vi "PH_ImageOperator.write PSDB Images data.vi"(0 "i ref in":refnum<vi>, 5 "error in":errorcluster) -> (14 "i ref out":refnum<vi>, 16 "Images Image data":T1[](array[typedef]), 17 "Images Boolean data":T3[](array[typedef]), 19 "error out":errorcluster)   [LabVIEW 2014, in "PH_ImageOperator.lvlib"]
uses:
  PH_ImageOperator.lvlib
  PH_Basics/PH_PSDBWriter/PH_PSDBWriter.Boolean dataset.ctl
  PH_Basics/PH_PSDBWriter/PH_PSDBWriter.Image dataset.ctl
  <vilib>/vision/Image Controls.llb/IMAQ Image.ctl
  <vilib>/vision/NI_Vision_Development_Module.lvlib
  PH_Basics/PH_PSDBWriter/PH_PSDBWriter.lvlib
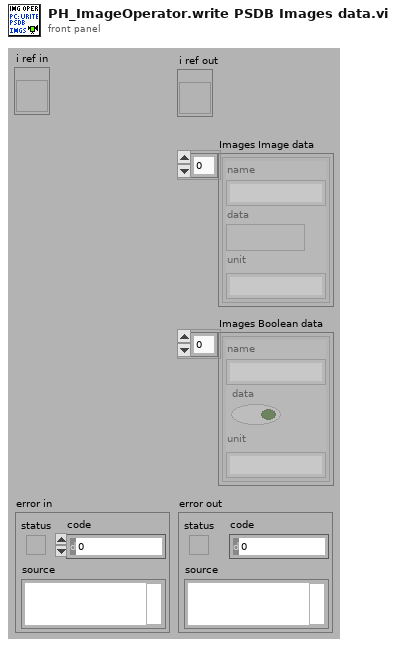
[diagram p1: front panel]
types:
  T1 = typedef "PH_PSDBWriter.lvlib/PH_PSDBWriter.Image dataset.ctl" = cluster{"name":string, "data":T2, "unit":string}
  T2 = typedef "IMAQ Image.ctl" = refnum<image>
  T3 = typedef "PH_PSDBWriter.lvlib/PH_PSDBWriter.Boolean dataset.ctl" = cluster{"name":string, "data":bool, "unit":string}
  T4 = typedef "Image Type" = u32
  T5 = typedef "PH_ImageOperator.lvlib/PH_ImageOperator.i attribute.ctl" = cluster{"GUI Refs":cluster{"Delete":refnum<vi>, "Calibration status":refnum<vi>, "BI subtracted":refnum<vi>, "calc Energy":refnum<vi>, "Energy: expected value":refnum<vi>, "Energy: Tolerance":refnum<vi>, "Energy calculated":refnum<vi>, "Energy":refnum<vi>, "calc Beam Anal":refnum<vi>, "Maj Diam 1/esquare":refnum<vi>, "Min Diam 1/esquare":refnum<vi>, "Azi Angle":refnum<vi>, "Min/Maj Diam esquare":refnum<vi>, "Beam analysed":refnum<vi>, "CoG - x":refnum<vi>, "CoG - y":refnum<vi>, "BA: Method":refnum<vi>, "BA: Steps":refnum<vi>, "BA: Factor":refnum<vi>, "calc Traces":refnum<vi>, "Traces: Fit Gauss":refnum<vi>, "Traces calculated":refnum<vi>, "Maj FWHM":refnum<vi>, "Min FWHM":refnum<vi>, "Major Trace":refnum<vi>, "Minor Trace":refnum<vi>, "Maj Fit Order":refnum<vi>, "Min Fit Order":refnum<vi>, "Position calculated":refnum<vi>, "Position":refnum<vi>, "Type":refnum<vi>, "Center":refnum<vi>, "exp - X":refnum<vi>, "exp - Y":refnum<vi>, "Tolerance":refnum<vi>, "f":refnum<vi>, "M":refnum<vi>, "D":refnum<vi>, "q":refnum<vi>, "Dummy Method":refnum<vi>, "Dummy Type":refnum<vi>, "Global On":refnum<vi>, "Traces: No offset":refnum<vi>, "Maj 99%":refnum<vi>, "Min 99%":refnum<vi>, "GUI FF Image":refnum<vi>, "calc Fill Factor":refnum<vi>, "FF calculated":refnum<vi>, "Fill Factor: Filter?":refnum<vi>, "FF: Damage Threshold":refnum<vi>, "FF: Threshold":refnum<vi>, "FF: max allow. Energy":refnum<vi>, "FF: Fillfactor":refnum<vi>, "Calibration data":refnum<vi>}, "List of GUIs":string[], "Calibration":cluster{"Status":T6, "Calibration data":T7, "Calibration Data File":path}, "Final Image":cluster{"BI Subtraction Failure":bool}, "Energy":cluster{"on":bool, "expected value [mJ]":dbl, "Tolerance [%]":dbl, "State":T6, "Energy [mJ]":dbl, "Unit":string, "calculated @":timestamp}, "Beam Analysis":cluster{"on":bool, "Data":T8, "Method":bool, "Steps":i32, "Factor":i32, "ROI":cluster{"Left":i32, "Top":i32, "Right":i32, "Bottom":i32}, "analysed @":timestamp}, "Trace Analysis":cluster{"on":bool, "Fit on":bool, "Maj FWHM":dbl, "Min FWHM":dbl, "Maj Fit Order":i32, "Min Fit Order":i32, "No Offset":bool, "Maj 99%":dbl, "Min 99%":dbl, "Traces":cluster{"XScaleName":string, "Y Scale Minimum":sgl, "Y Scale Maximum":sgl, "X Scale Minimum":sgl, "X Scale Maximum":sgl, "Traces":cluster{"Index":sgl[], "Trace":dbl[]}[]}[], "analysed @":timestamp}, "Position Analysis":cluster{"on":bool, "exp - X":i32, "exp - Y":i32, "focal length [mm]":dbl, "Magnification":dbl, "Delta":dbl, "Theta":dbl, "Tolerance":dbl, "Type":bool, "analysed @":timestamp}, "Fill Factor":cluster{"on":bool, "Filter on?":bool, "Threshold":dbl, "Damage Threshold [J/cm²]":dbl, "Fillfactor":dbl, "Max. allowed Energy [J]":dbl, "calculated @":timestamp}, "Statistician Service ID":i32, "Images":cluster{"Background":T2, "OP":T2, "GUI":T2, "BA: ROI":T2, "Trace: Turn":T2, "FF: Main":T2, "FF: Help":T2, "PSDB: BG":T2, "PSDB: OP":T2, "PSDB: FF":T2}}
  T6 = typedef "PH_StatusHandler.lvlib/PH_StatusHandler.Status.ctl" = i16
  T7 = typedef "PH_ImageCalibrator.lvlib/PH_ImageCalibrator.Calibration Data.ctl" = cluster{"Date":string, "Time":string, "Cam Settings":cluster{"Cam ID":string, "Gain":dbl, "Brightness":dbl, "Shutter":dbl, "Cam Error":bool, "Mode":i32}, "Background Image":cluster{"Image":dbl[][], "Image Error":bool}, "Linear Calibration":cluster{"Calibration Factor":dbl, "not mm or mrad":bool}, "Energy Calibration":cluster{"Calibration Factor":dbl, "no mJ":bool}}
  T8 = typedef "PH_ImageOperator.lvlib/PH_ImageOperator.Beam Analysis Data.ctl" = cluster{"CoG-x":sgl, "CoG-y":sgl, "Maj Dim":dbl, "Min Dim":dbl, "Ellipticity":dbl, "Azimuth Angle [rad]":dbl, "Azi Angle rel to Maj?":bool}
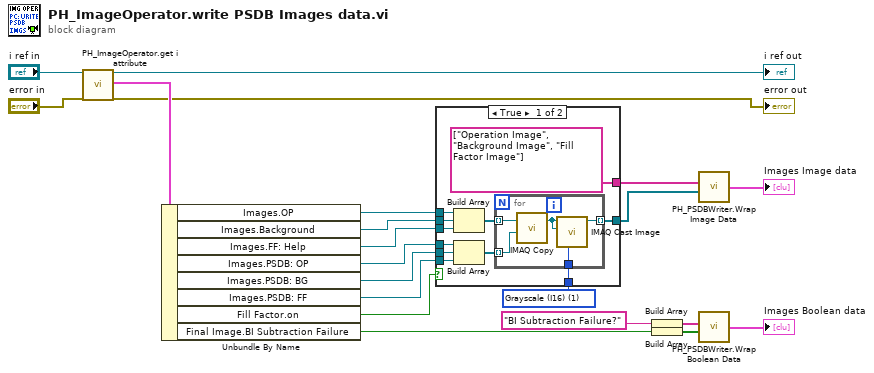
[diagram p0: block diagram]
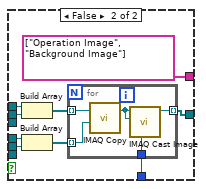
[diagram p2: hidden frame]
diagram:
  w6 = T4 1 items=["Grayscale (U8)", "Grayscale (I16)", "Grayscale (SGL)", "Complex (CSG)", "RGB (U32)", "HSL (U32)", "RGB (U64)", "Grayscale (U16)"] ("Image Type")
  n1 = call "PH_ImageOperator.get i attribute.vi"("i ref in"="i ref in", "error in (no error)"="error in") -> ("i ref out"=→"i ref out":refnum<vi>, "i attribute"=w21:T5, "error out"=→"error out":errorcluster)  [unwired: 15 in]
  n2 = Unbundle By Name(w21) -> ("Images.OP"=w12:T2, "Images.Background"=w11:T2, "Images.FF: Help"=w10:T2, "Images.PSDB: OP"=w9:T2, "Images.PSDB: BG"=w8:T2, "Images.PSDB: FF"=w7:T2, "Fill Factor.on"=w13:bool, "Final Image.BI Subtraction Failure"=w4:bool)
  n3 = case shown="True" w13 {
    tunnel: w11 -> [w30 w44]
    tunnel: w12 -> [w31 w45]
    tunnel: [string[] ["Operation Image", "Background Image", "Fill Factor Image"] string[] ["Operation Image", "Background Image"]] -> w16
    tunnel: [w23 w39] -> w14
    tunnel: w10 -> [w29 _]
    tunnel: w9 -> [w28 w41]
    tunnel: w8 -> [w27 w40]
    tunnel: w7 -> [w26 _]
    tunnel: w6 -> [w22 w38]
    frame True {
      n4 = Build Array(w31, w30, w29) -> (w25:T2[])
      n5 = Build Array(w28, w27, w26) -> (w24:T2[])
      n6 = for {
        tunnel: w25 -> [w34] mode=indexing
        tunnel: w24 -> [w35] mode=indexing
        tunnel: [w37] -> w23 mode=indexing
        tunnel: w22 -> [w36]
        n7 = call "IMAQ Copy"("Image Dst"=w35, "Image Src"=w34) -> ("Image Dst Out"=w33:T2)  [unwired: 4 in, 1 out]
        n8 = call "IMAQ Cast Image"("Image Type"=w36, "Image Dst"=w33, "Image Src"=w33) -> ("Image Dst Out"=w37:T2)  [unwired: 7 in, 1 out]
      }
    }
    frame False {
      n9 = Build Array(w45, w44) -> (w43:T2[])
      n10 = Build Array(w41, w40) -> (w42:T2[])
      n11 = for {
        tunnel: w43 -> [w48] mode=indexing
        tunnel: w42 -> [w49] mode=indexing
        tunnel: [w51] -> w39 mode=indexing
        tunnel: w38 -> [w50]
        n12 = call "IMAQ Copy"("Image Dst"=w49, "Image Src"=w48) -> ("Image Dst Out"=w47:T2)  [unwired: 4 in, 1 out]
        n13 = call "IMAQ Cast Image"("Image Type"=w50, "Image Dst"=w47, "Image Src"=w47) -> ("Image Dst Out"=w51:T2)  [unwired: 7 in, 1 out]
      }
    }
  }
  n14 = Build Array("BI Subtraction Failure?" ("string")) -> (w2:string[])
  n15 = Build Array(w4) -> (w1:bool[])
  n16 = call "PH_PSDBWriter.Wrap Image Data.vi"("Data Arrray"=w14, "Name Array"=w16) -> ("PSDB Image Data Array"=→"Images Image data":T1[])  [unwired: 2 in]
  n17 = call "PH_PSDBWriter.Wrap Boolean Data.vi"("Data Array"=w1, "Name Array"=w2) -> ("PSDB Boolean Data Array"=→"Images Boolean data":T3[])  [unwired: 2 in]
